vi "Add to Array if Not Present (DBL).vi"(4 "DBL":dbl, 5 "DBL Array":dbl[](array[numeric])) -> (1 "New DBL Array":dbl[](array[numeric]))   [LabVIEW 2011]
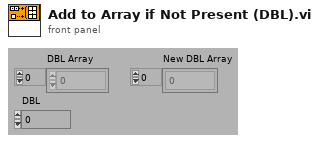
[diagram p1: front panel]
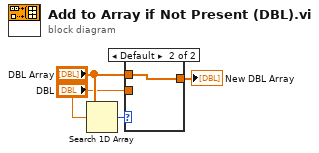
[diagram p0: block diagram]
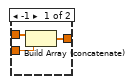
[diagram p2: hidden frame]
diagram:
  n1 = Search 1D Array(1D array="DBL Array", element="DBL") -> (index of element=w4:i32)  [unwired: 1 out]
  n2 = case shown="Default" w4 {
    tunnel: "DBL Array" -> [w7 w8]
    tunnel: "DBL" -> [w6 _]
    tunnel: [w5 w8] -> w1
    frame -1 {
      n3 = Build Array (concatenate)(w7, w6) -> (w5:dbl[])
    }
    frame Default {
    }
  }
  "New DBL Array" <- w1
